vi "Enable_Disable Single.vi"(8 "error in (no error)":errorcluster, 9 "Enable (T)":bool, 10 "Control Name":string, 11 "Controls_Mgr in":refnum<class "Controls_Mgr.lvclass">) -> (0 "error out":errorcluster, 3 "Controls_Mgr out":refnum<class "Controls_Mgr.lvclass">)   [LabVIEW 2015, in "Generic Module Library.lvlib" / "Template G_Module.lvlib" / "Controls_Mgr.lvclass"]
uses:
  Controls_Mgr.lvclass
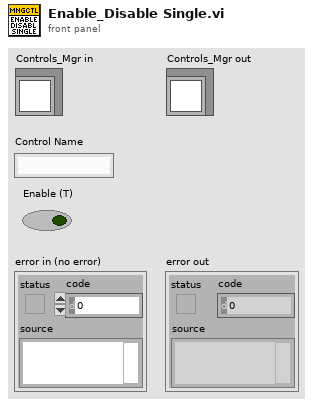
[diagram p1: front panel]
types:
  T1 = enum8{"Enabled", "Disabled", "Disabled and Grayed Out"}
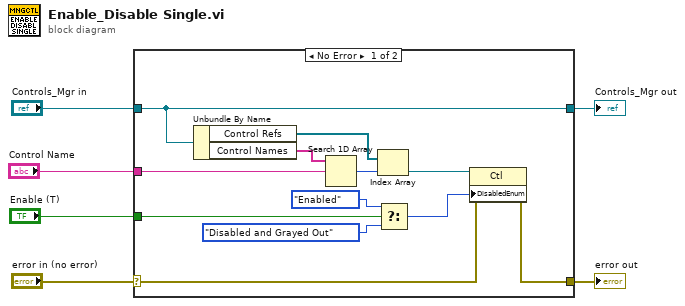
[diagram p0: block diagram]
diagram:
  n1 = case shown="No Error" "error in (no error)" {
    selector: "error in (no error)" -> [w8 w20]
    tunnel: [w7 w20] -> w5
    tunnel: [w15 w19] -> w3
    tunnel: "Controls_Mgr in" -> [w15 w19]
    tunnel: "Control Name" -> [w14 _]
    tunnel: "Enable (T)" -> [w12 _]
    frame No Error {
      n2 = Unbundle By Name(w15) -> ("Control Refs"=w16:refnum<vi>[], "Control Names"=w18:string[])
      n3 = Search 1D Array(1D array=w18, element=w14) -> (index of element=w17:i32)  [unwired: 1 in]
      n4 = Index Array(array=w16, index=w17) -> (element=w13:refnum<vi>)
      n5 = Select(t=T1."Enabled" ("Disabled"), s=w12, f=T1."Disabled and Grayed Out" ("Disabled")) -> (s? t:f=w9:T1)
      n6 = property class="Ctl"(reference=w13, error in=w8, "DisabledEnum"=w9) -> (error out=w7:errorcluster)  [unwired: 1 out]
    }
    frame Error {
    }
  }
  "error out" <- w5
  "Controls_Mgr out" <- w3
